vi "test_LongRecording.vi"() -> ()   [LabVIEW 2011]
uses:
  <vilib>/Platform/TimedLoop/XDataNode/timing_clust.ctl
  <vilib>/Platform/TimedLoop/XDataNode/nitl_modes.ctl
  <vilib>/Platform/TimedLoop/XDataNode/wakeup.ctl
  <vilib>/Platform/TimedLoop/XDataNode/XDataNode.xnode
  <vilib>/Platform/TimedLoop/XDataNode/XDNodeRunTimeDep.lvlib
  <vilib>/vision/NI_Vision_Development_Module.lvlib
panel:
  in  "名称或相对路径":string="Test01.blk"
  in  "停止":bool
  out "Y Resolution":i32
  out "X Resolution":i32
  in  "datatype":enum16{"U8", "I16", "U32", "SGL"}(ring)=enum."SGL"
  in  "Recording":bool
  in  "BlkFolderPath":path=path "C:/Documents and Settings/VdaqUser/Desktop/imager for flowbit/testBLK"
  out "当前blk句柄":refnum<file>
  out "循环持续时间":i64
  out "Image":T1(plugin-control)
  in  "热图":bool
  in  "bin_num":i32=25
  out "队列中元素数量":i32(slide) scale=0.0..100.0
  in  "frame_count":i32
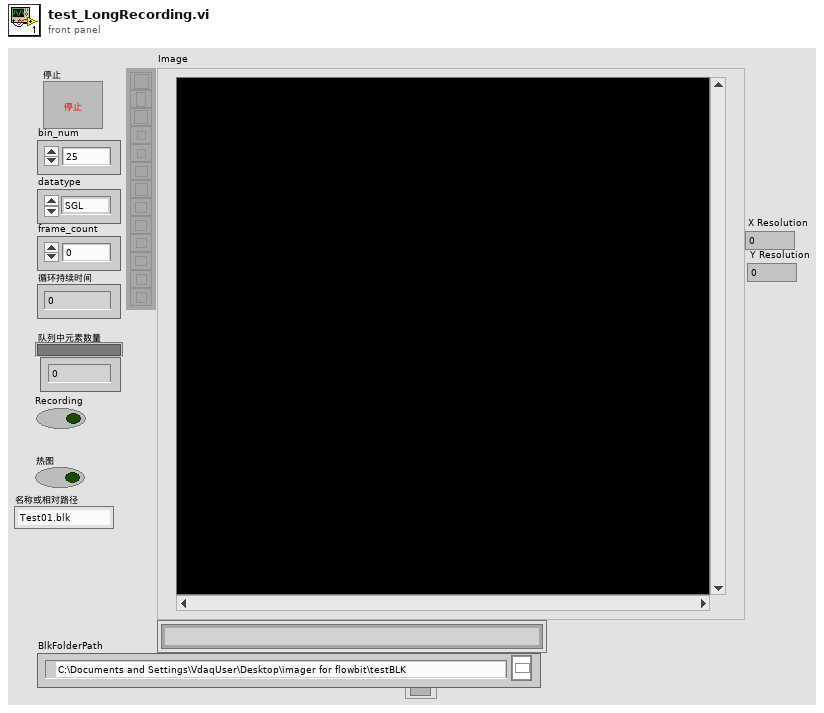
[diagram p1: front panel]
types:
  T1 = typedef "IMAQ Image.ctl" = refnum<image>
  T2 = typedef "Image Type" = u32
  T3 = enum16{"Disable External Trigger", "Enable External Trigger"}
  T4 = enum32{"Auto Detect", "RoadRunner", "Raven", "R64"}
  T5 = enum16{"open", "replace", "create", "open or create", "replace or create", "replace or create with confirmation"}
  T6 = typedef "XDNodeRunTimeDep.lvlib/timing_clust.ctl" = cluster{"Expected End [f-1]":u64, "Actual End [f-1]":u64, "Finished Late? [f-1]":bool, "Expected End [i-1]":u64, "Actual End [i-1]":u64, "Finished Late? [i-1]":bool, "Expected Start [i]":u64, "Actual Start [i]":u64, "Expected Start [f]":u64, "Actual Start [f]":u64, "Source Name":string, "Structure Name":string, "Period":i64, "Deadline":i64, "Offset":i64, "Start":i64, "Priority":i32, "Timeout":i32, "Mode":T7, "Wakeup Reason":T8, "Error":errorcluster, "Source Type":string, "Secondary Source Type":string, "Global End Time":u64, "Global Start Time":u64, "Frame Duration":u64, "Iteration Duration":u64, "Assigned CPU":i32, "I/O Scan Engine Mode":u32}
  T7 = typedef "XDNodeRunTimeDep.lvlib/nitl_modes.ctl" = enum32{"No Change", "Process missed periods, maintain original phase", "Discard missed periods, maintain original phase", "Process missed periods, ignore original phase", "Discard missed periods, ignore original phase"}
  T8 = typedef "XDNodeRunTimeDep.lvlib/wakeup.ctl" = enum32{"Normal", "Aborted", "Asynchronous wakeup", "Timing source error", "Timed loop error", "Timeout"}
  T9 = enum16{"big-endian, network order", "native, host order", "little-endian"}
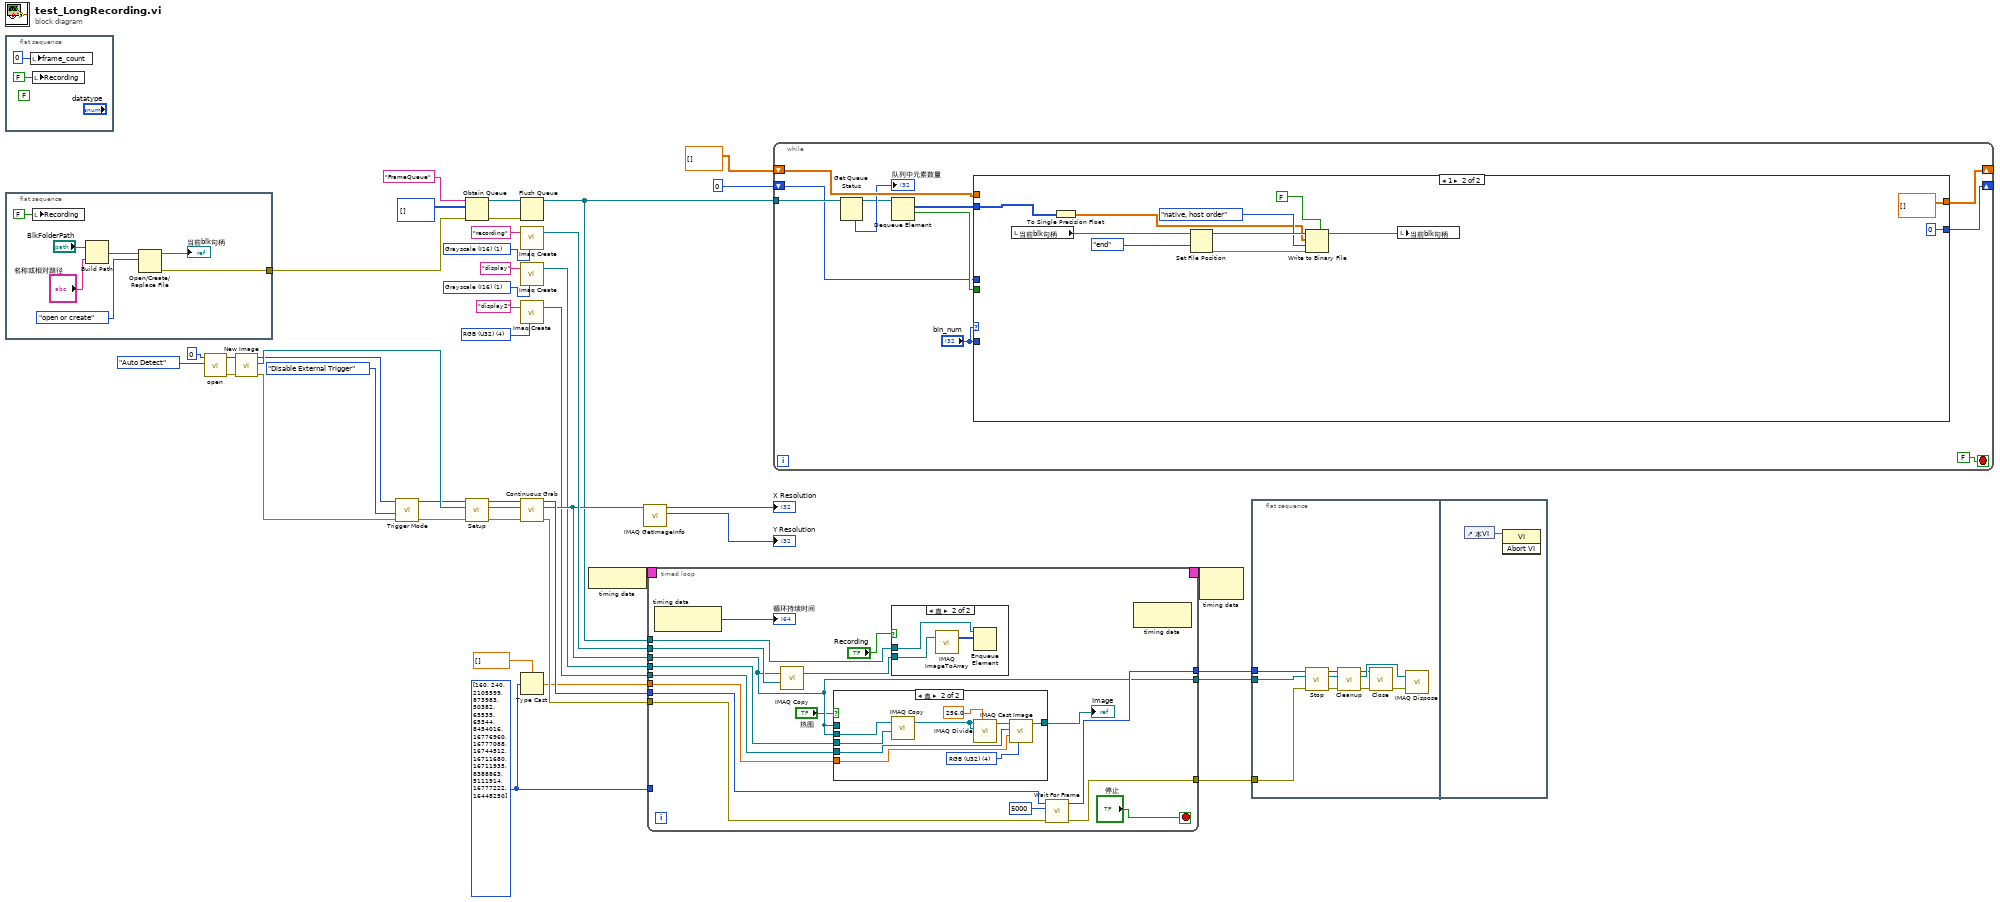
[diagram p0: block diagram]
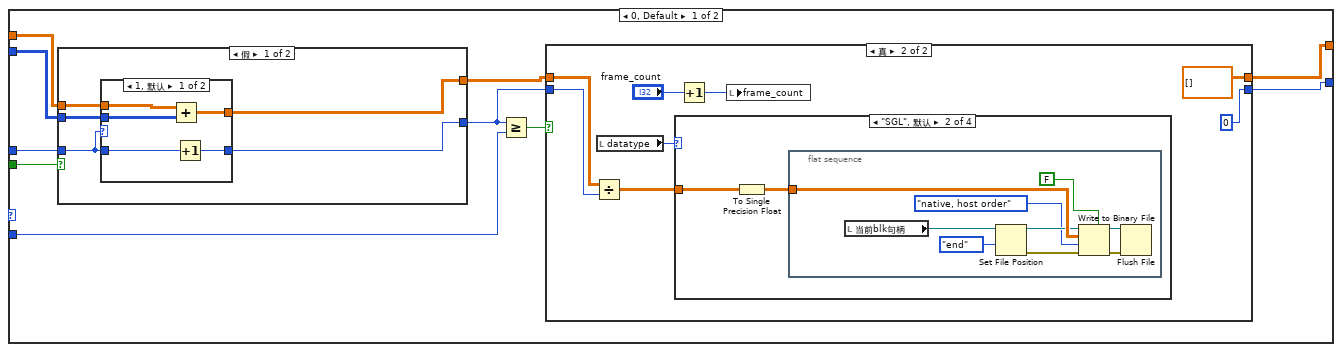
[diagram p2: hidden frame]
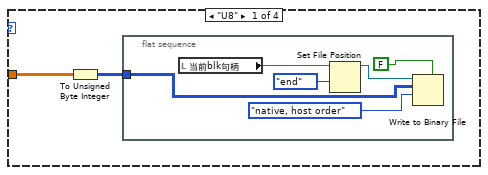
[diagram p4: hidden frame]
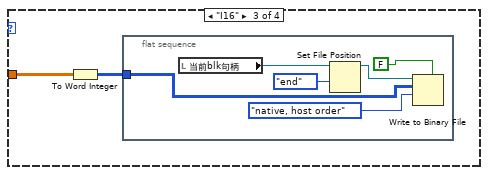
[diagram p5: hidden frame]
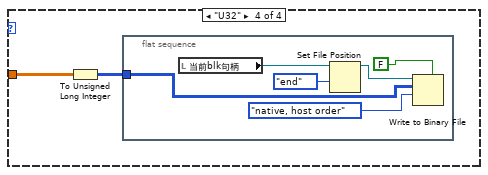
[diagram p6: hidden frame]
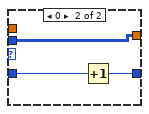
[diagram p7: hidden frame]
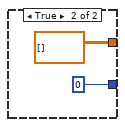
[diagram p8: hidden frame]
diagram:
  w7 = T2 4 items=["Grayscale (U8)", "Grayscale (I16)", "Grayscale (SGL)", "Complex (CSG)", "RGB (U32)", "HSL (U32)", "RGB (U64)", "Grayscale (U16)"] ("Image Type")
  w5 = u32[] [160, 240, 2105599, 873983, 50382, 65535, 65344, 8454016, 16776960, 16777088, 16744512, 16711680, 16711935, 8388863, 5111914, 16777222, 16448250] ("数组")
  w11 = T2 1 items=["Grayscale (U8)", "Grayscale (I16)", "Grayscale (SGL)", "Complex (CSG)", "RGB (U32)", "HSL (U32)", "RGB (U64)", "Grayscale (U16)"] ("Image Type")
  w21 = T2 1 items=["Grayscale (U8)", "Grayscale (I16)", "Grayscale (SGL)", "Complex (CSG)", "RGB (U32)", "HSL (U32)", "RGB (U64)", "Grayscale (U16)"] ("Image Type")
  n1 = flat-sequence {
    frame #0 {
      (unwired) FALSE ("停止 3")
      n2 = local write "frame_count"(0 ("frame_count")) -> ()
      n3 = local write "Recording"(FALSE ("Recording")) -> ()
    }
  }
  n4 = flat-sequence {
    tunnel: [w46] -> w2
    frame #0 {
      n5 = local write "Recording"(FALSE ("Recording")) -> ()
      n6 = Build Path(base path="BlkFolderPath", name or relative path="名称或相对路径") -> (appended path=w50:path)
      n7 = Open/Create/Replace File(file path (use dialog)=w50, operation (0:open)=T5."open or create" ("操作(0:open)")) -> (refnum out=→"当前blk句柄":refnum<file>, error out=w46:errorcluster)  [unwired: 4 in, 1 out]
    }
  }
  n8 = call <vilib>:"open.vi"("Board Type"=T4."Auto Detect", "Board Number"=u32 0) -> ("error out"=w34:errorcluster, "RefBrdOut"=w29:u32)  [unwired: 2 in, 5 out]
  n9 = call <vilib>:"New Image.vi"("RefBrdIn"=w29, "error in"=w34) -> ("RefBrdOut"=w28:u32, "Image"=w39:T1, "error out"=w35:errorcluster)  [unwired: 6 in]
  n10 = call <vilib>:"Trigger Mode.vi"("RefBrdIn"=w28, "Trigger Mode"=T3."Disable External Trigger", "error in (no error)"=w35) -> ("RefBrdOut"=w27:u32, "error out"=w36:errorcluster)  [unwired: 6 in]
  n11 = Obtain Queue(name (unnamed)="FrameQueue" ("名称（未命名）"), element data type=i16[][] [], error in (no error)=w2) -> (queue out=w13:refnum<queue>, error out=w1:errorcluster)  [unwired: 2 in, 1 out]
  n12 = call <vilib>:"Setup.vi"("error in"=w36, "Image In"=w39, "RefBrdIn"=w27) -> ("error out"=w31:errorcluster, "Image"=w32:T1, "RefBrdOut"=w26:u32)  [unwired: 6 in]
  n13 = Flush Queue(queue=w13, error in (no error)=w1) -> (queue out=w12:refnum<queue>)  [unwired: 2 out]
  n14 = call "Imaq Create"("Image Name"="recording", "Image Type"=w21) -> ("New Image"=w23:T1)  [unwired: 3 in, 1 out]
  n15 = call "Imaq Create"("Image Name"="display", "Image Type"=w11) -> ("New Image"=w9:T1)  [unwired: 3 in, 1 out]
  n16 = call "Imaq Create"("Image Name"="display2", "Image Type"=w7) -> ("New Image"=w6:T1)  [unwired: 3 in, 1 out]
  n17 = call <vilib>:"Continuous Grab.vi"("error in (no error)"=w31, "Image In"=w32, "RefBrdIn"=w26) -> ("error out"=w30:errorcluster, "Image"=w16:T1, "RefBrdOut"=w25:u32)  [unwired: 6 in]
  n18 = Type Cast(type=sgl[] [] ("单精度浮点"), x=w5) -> (*(type *) &x=w3:sgl[])
  n19 = node-c288() -> (w43:T6)
  n20 = call "IMAQ GetImageInfo"("Image"=w16) -> ("Y Resolution"=→"Y Resolution":i32, "X Resolution"=→"X Resolution":i32)  [unwired: 3 in, 6 out]
  n21 = timed-loop {
    tunnel: [w57] -> w38
    tunnel: [w69] -> w37
    tunnel: w16 -> [w57]
    tunnel: w30 -> [w68]
    tunnel: w25 -> [w67]
    tunnel: [w66] -> w24
    timing: w43 -> [_]
    timing-out: [_] -> w42
    tunnel: w23 -> [w62]
    tunnel: w12 -> [w64]
    tunnel: w9 -> [w60]
    tunnel: w5 -> [_]
    tunnel: w6 -> [w59]
    tunnel: w3 -> [w58]
    stop <- "停止" stop-if-true
    n22 = node-c288() -> (→"循环持续时间":i64)  [unwired: 1 in]
    n23 = call "IMAQ Copy"("Image Dst"=w62, "Image Src"=w57) -> ("Image Dst Out"=w61:T1)  [unwired: 4 in, 1 out]
    n24 = case shown="真" "热图" {
      tunnel: w60 -> [_ w78]
      tunnel: w57 -> [_ w76]
      tunnel: [w70 w75] -> w56
      tunnel: w59 -> [_ w73]
      tunnel: w58 -> [_ w72]
      tunnel: w57 -> [w70 _]
      frame False {
      }
      frame True {
        w74 = T2 4 items=["Grayscale (U8)", "Grayscale (I16)", "Grayscale (SGL)", "Complex (CSG)", "RGB (U32)", "HSL (U32)", "RGB (U64)", "Grayscale (U16)"] ("Image Type")
        n25 = call "IMAQ Copy"("Image Dst"=w78, "Image Src"=w76) -> ("Image Dst Out"=w77:T1)  [unwired: 4 in, 1 out]
        n26 = call "IMAQ Divide"("Image Src A"=w77, "Constant"=sgl 256.0, "Image Dst"=w77) -> ("Image Dst Out"=w71:T1)  [unwired: 4 in, 1 out]
        n27 = call "IMAQ Cast Image"("Image Type"=w74, "Lookup Table"=w72, "Image Dst"=w73, "Image Src"=w71) -> ("Image Dst Out"=w75:T1)  [unwired: 6 in, 1 out]
      }
    }
    "Image" <- w56
    n28 = case shown="真" "Recording" {
      tunnel: w64 -> [_ w80]
      tunnel: w61 -> [_ w82]
      frame False {
      }
      frame True {
        n29 = call "IMAQ ImageToArray"("Image"=w82) -> ("Image Pixels (I16)"=w81:i16[][])  [unwired: 3 in, 4 out]
        n30 = Enqueue Element(queue=w80, element=w81) -> ()  [unwired: 2 in, 3 out]
      }
    }
    n31 = call <vilib>:"Wait For Frame.vi"("error in (no error)"=w68, "Timeout (mS)"=u32 5000, "RefBrdIn"=w67) -> ("error out"=w69:errorcluster, "RefBrdOut"=w66:u32)  [unwired: 7 in]
    n32 = node-c288() -> ()  [unwired: 1 in, 1 out]
  }
  n33 = while {
    tunnel: w12 -> [w96]
    shift-right: [w91] -> _
    shift-left: sgl[][] [] -> [w93]
    shift-right: [w90] -> _
    shift-left: 0 ("加法记数") -> [w92]
    stop <- FALSE stop-if-true
    n34 = Get Queue Status(queue=w96) -> (queue out=w88:refnum<queue>, # elements in queue=→"队列中元素数量":i32)  [unwired: 2 in, 6 out]
    n35 = Dequeue Element(queue=w88) -> (element=w94:i16[][], timed out?=w95:bool)  [unwired: 2 in, 2 out]
    n36 = case shown="1" "bin_num" {
      tunnel: w95 -> [w106 _]
      tunnel: w94 -> [w105 w169]
      tunnel: w93 -> [w104 _]
      tunnel: w92 -> [w103 _]
      tunnel: "bin_num" -> [w101 _]
      tunnel: [w100 sgl[][] []] -> w91
      tunnel: [w99 0 ("加法记数")] -> w90
      frame 0, Default {
        n37 = case shown="假" w106 {
          tunnel: w105 -> [w156 _]
          tunnel: [w155 sgl[][] []] -> w102
          tunnel: w104 -> [w154 _]
          tunnel: w103 -> [w153 _]
          tunnel: [w152 0] -> w98
          frame False {
            n38 = case shown="1, 默认" w153 {
              tunnel: w156 -> [w161 w164]
              tunnel: [w159 w164] -> w155
              tunnel: w154 -> [w160 _]
              tunnel: w153 -> [w158 w163]
              tunnel: [w157 w162] -> w152
              frame 1, Default {
                n39 = Add(x=w160, y=w161) -> (x+y=w159:sgl[][])
                n40 = Increment(x=w158) -> (x+1=w157:i32)
              }
              frame 0 {
                n41 = Increment(x=w163) -> (x+1=w162:i32)
              }
            }
          }
          frame True {
          }
        }
        n42 = Greater Or Equal?(x=w98, y=w101) -> (x >= y?=w97:bool)
        n43 = case shown="真" w97 {
          tunnel: w102 -> [w108 w115]
          tunnel: [w108 sgl[][] []] -> w100
          tunnel: w98 -> [w107 w113]
          tunnel: [w107 0 ("加法记数")] -> w99
          frame False {
          }
          frame True {
            n44 = Divide(x=w115, y=w113) -> (x/y=w116:sgl[][])
            n45 = local read "datatype"() -> (w109:enum16{"U8", "I16", "U32", "SGL"})
            n46 = case shown="\"SGL\", 默认" w109 {
              tunnel: w116 -> [w118 w126 w137 w145]
              frame "U8" {
                n47 = To Unsigned Byte Integer(number=w118) -> (unsigned 8bit integer=w117:u8[][])
                n48 = flat-sequence {
                  tunnel: w117 -> [w123]
                  frame #0 {
                    n49 = local read "当前blk句柄"() -> (w124:refnum<file>)
                    n50 = Set File Position(refnum=w124, from (0:start)=enum16{"start", "end", "current"}."end" ("自（0:起始）")) -> (refnum out=w122:refnum<file>)  [unwired: 2 in, 1 out]
                    n51 = Write to Binary File(file (use dialog)=w122, data=w123, 5:FALSE ("预置数组或字符串大小？(T)"), 9:T9."native, host order" ("字节顺序(0:big-endian, network order)")) -> ()  [unwired: 2 in, 3 out]
                  }
                }
              }
              frame "SGL", Default {
                n52 = To Single Precision Float(number=w126) -> (single precision float=w125:sgl[][])
                n53 = flat-sequence {
                  tunnel: w125 -> [w134]
                  frame #0 {
                    n54 = local read "当前blk句柄"() -> (w135:refnum<file>)
                    n55 = Set File Position(refnum=w135, from (0:start)=enum16{"start", "end", "current"}."end" ("自（0:起始）")) -> (refnum out=w133:refnum<file>, error out=w127:errorcluster)  [unwired: 2 in]
                    n56 = Write to Binary File(file (use dialog)=w133, data=w134, error in=w127, 5:FALSE ("预置数组或字符串大小？(T)"), 9:T9."native, host order" ("字节顺序(0:big-endian, network order)")) -> (refnum out=w129:refnum<file>, error out=w128:errorcluster)  [unwired: 1 in, 1 out]
                    n57 = Flush File(refnum=w129, error in=w128) -> ()  [unwired: 2 out]
                  }
                }
              }
              frame "I16" {
                n58 = To Word Integer(number=w137) -> (16bit integer=w136:i16[][])
                n59 = flat-sequence {
                  tunnel: w136 -> [w142]
                  frame #0 {
                    n60 = local read "当前blk句柄"() -> (w143:refnum<file>)
                    n61 = Set File Position(refnum=w143, from (0:start)=enum16{"start", "end", "current"}."end" ("自（0:起始）")) -> (refnum out=w141:refnum<file>)  [unwired: 2 in, 1 out]
                    n62 = Write to Binary File(file (use dialog)=w141, data=w142, 5:FALSE ("预置数组或字符串大小？(T)"), 9:T9."native, host order" ("字节顺序(0:big-endian, network order)")) -> ()  [unwired: 2 in, 3 out]
                  }
                }
              }
              frame "U32" {
                n63 = To Unsigned Long Integer(number=w145) -> (unsigned 32bit integer=w144:u32[][])
                n64 = flat-sequence {
                  tunnel: w144 -> [w150]
                  frame #0 {
                    n65 = local read "当前blk句柄"() -> (w151:refnum<file>)
                    n66 = Set File Position(refnum=w151, from (0:start)=enum16{"start", "end", "current"}."end" ("自（0:起始）")) -> (refnum out=w149:refnum<file>)  [unwired: 2 in, 1 out]
                    n67 = Write to Binary File(file (use dialog)=w149, data=w150, 5:FALSE ("预置数组或字符串大小？(T)"), 9:T9."native, host order" ("字节顺序(0:big-endian, network order)")) -> ()  [unwired: 2 in, 3 out]
                  }
                }
              }
            }
            n68 = Increment(x="frame_count") -> (x+1=w110:i32)
            n69 = local write "frame_count"(w110) -> ()
          }
        }
      }
      frame 1 {
        n70 = local read "当前blk句柄"() -> (w175:refnum<file>)
        n71 = To Single Precision Float(number=w169) -> (single precision float=w168:sgl[][])
        n72 = Set File Position(refnum=w175, from (0:start)=enum16{"start", "end", "current"}."end" ("自（0:起始）")) -> (refnum out=w174:refnum<file>, error out=w170:errorcluster)  [unwired: 2 in]
        n73 = Write to Binary File(file (use dialog)=w174, data=w168, error in=w170, 5:FALSE ("预置数组或字符串大小？(T)"), 9:T9."native, host order" ("字节顺序(0:big-endian, network order)")) -> (refnum out=w167:refnum<file>)  [unwired: 1 in, 2 out]
        n74 = local write "当前blk句柄"(w167) -> ()
      }
    }
  }
  n75 = node-c288(w42) -> ()  [unwired: 1 out]
  n76 = flat-sequence {
    tunnel: w38 -> [w187]
    tunnel: w37 -> [w182]
    tunnel: w24 -> [w181]
    frame #0 {
      n77 = call <vilib>:"Stop.vi"("error in (no error)"=w182, "Image In"=w187, "RefBrdIn"=w181) -> ("error out"=w183:errorcluster, "Image"=w186:T1, "RefBrdOut"=w180:u32)  [unwired: 6 in]
      n78 = call <vilib>:"Cleanup.vi"("error in (no error)"=w183, "Image In"=w186, "RefBrdIn"=w180) -> ("error out"=w184:errorcluster, "Image"=w185:T1, "RefBrdOut"=w179:u32)  [unwired: 6 in]
      n79 = call <vilib>:"Close.vi"("error in (no error)"=w184, "RefBrdIn"=w179) -> ("error out"=w178:errorcluster)  [unwired: 8 in, 1 out]
      n80 = call "IMAQ Dispose"("Image"=w185, "error in (no error)"=w178) -> ()  [unwired: 4 in, 1 out]
    }
    frame #1 {
      n81 = control-ref of="本VI"() -> (w188:refnum<vi>)
      n82 = invoke class="VI" method="Abort VI"(reference=w188) -> ()  [unwired: 2 in, 3 out]
    }
  }
